vi "After.vi"(8 "Error In":errorcluster, 10 "Remote Source Path":string, 11 "SFTP In":refnum<class "SFTP.lvclass">) -> (0 "Error Out":errorcluster, 3 "Session Out":refnum<class "Session.lvclass">)   [LabVIEW 2018, in "Tests.lvlib" / "SFTP.lvlib"]
uses:
  SFTP.lvlib
  src/Toolkit/API/SFTP/SFTP.lvclass
  src/Toolkit/API/Session/Session.lvclass
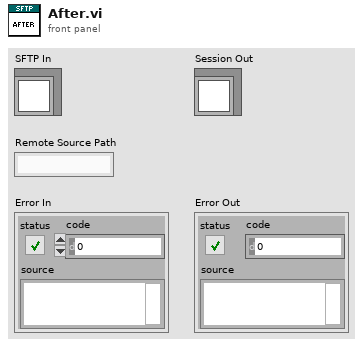
[diagram p1: front panel]
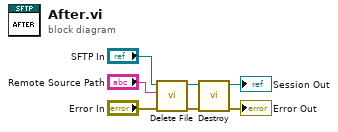
[diagram p0: block diagram]
diagram:
  n1 = call "Delete File.vi"("Error In"="Error In", "Remote Path"="Remote Source Path", "SFTP In"="SFTP In") -> ("Error Out"=w6:errorcluster, "SFTP Out"=w5:refnum<class "SFTP.lvclass">)  [unwired: 7 in]
  n2 = call "Destroy.vi"("Error In"=w6, "SFTP"=w5) -> ("Error Out"=→"Error Out":errorcluster, "Session"=→"Session Out":refnum<class "Session.lvclass">)  [unwired: 8 in]
